vi "Get Image Pointer.vi"(8 "error in (no error)":errorcluster, 10 "Image Data":variant, 11 "Image in":T1) -> (0 "error out":errorcluster, 2 "Loaded Image Data (float)":sgl[][](array[numeric]), 3 "Image out":T1)   [LabVIEW 2011, in "Meter Detection Custom Device.lvlib"]
uses:
  <vilib>/vision/Image Controls.llb/IMAQ Image.ctl
  Meter Detection Custom Device.lvlib
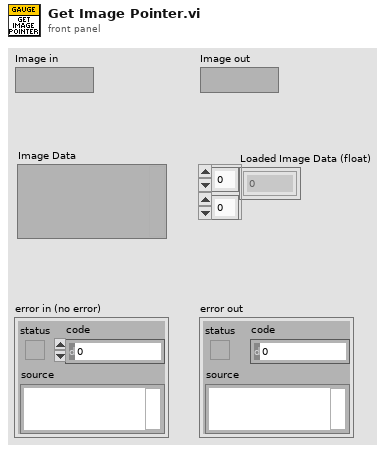
[diagram p1: front panel]
types:
  T1 = typedef "IMAQ Image.ctl" = refnum<image>
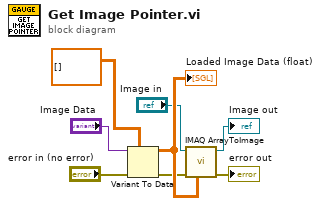
[diagram p0: block diagram]
diagram:
  n1 = Variant To Data(error in="error in (no error)", type=sgl[][] [] ("Image Pixels (I16)"), Variant="Image Data") -> (data=w7:sgl[][], error out=w4:errorcluster)
  "Loaded Image Data (float)" <- w7
  n2 = call "IMAQ ArrayToImage"("Image Pixels (Float)"=w7, "error in (no error)"=w4, "Image"="Image in") -> ("error out"=→"error out":errorcluster, "Image Out"=→"Image out":T1)  [unwired: 7 in]
